vi "Floating Panel.vi"(11 "VI Refnum":refnum<vi>) -> ()   [LabVIEW 2009, in "UI Panels.lvlib" / "Panels_XControl.xctl"]
uses:
  Panels_XControl.xctl
panel:
  in  "Dock Feedback":refnum<user-event>
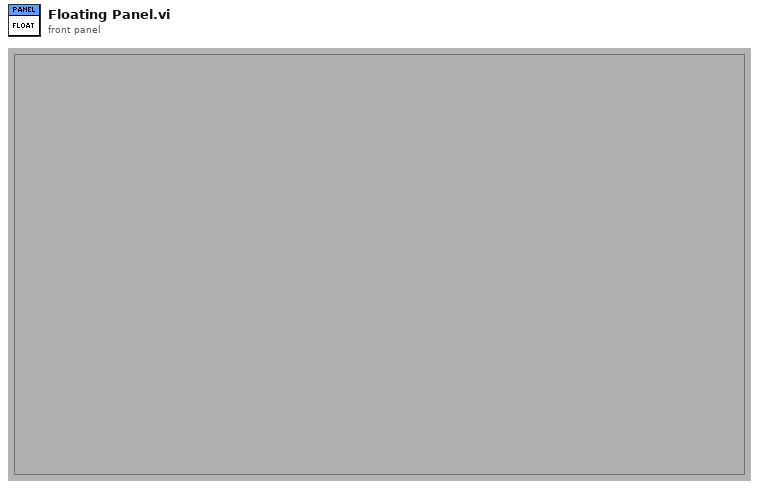
[diagram p1: front panel]
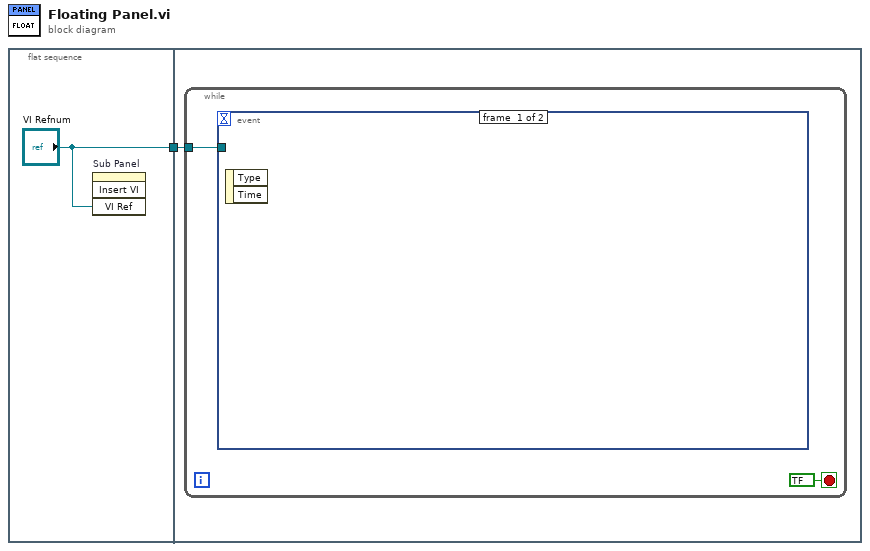
[diagram p0: block diagram]
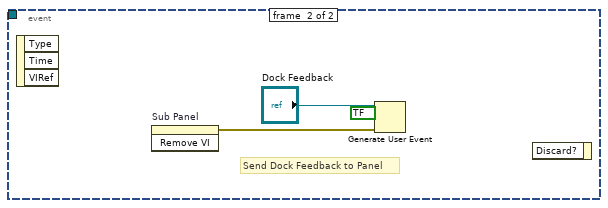
[diagram p2: hidden frame]
diagram:
  n1 = flat-sequence {
    tunnel: ["VI Refnum"] -> w1
    tunnel: w1 -> [w3]
    frame #0 {
      n2 = invoke on="Sub Panel" class="SubPanel" method="Insert VI"("VI Ref"="VI Refnum") -> ()  [unwired: 3 in, 4 out]
    }
    frame #1 {
      n3 = while {
        tunnel: w3 -> [w4]
        stop <- bool ? stop-if-true
        n4 = event shown="[1] Panel Close?" {
          selector: _ -> [_ _]
          dyn-events: _ -> [_ _]
          timeout: _ -> [_ _]
          tunnel: w4 -> [_ _]
          event #0 {
            n5 = event-data() -> ()  [unwired: 1 in, 2 out]
          }
          event #1 {
            # "Send Dock Feedback to Panel"
            n6 = event-data() -> ()  [unwired: 1 in, 3 out]
            n7 = invoke on="Sub Panel" class="SubPanel" method="Remove VI"() -> (error out=w6:errorcluster)  [unwired: 3 in, 2 out]
            n8 = Generate User Event(user event="Dock Feedback", event data cluster=bool ? ("event data"), error in=w6) -> ()  [unwired: 2 out]
            n9 = event-data() -> ()  [unwired: 2 in, 1 out]
          }
        }
      }
    }
  }
